vi "AddNextNode.vi"(8 "error in (no error)":errorcluster, 10 "Palette Name(Next)":string, 11 "VI Ref":refnum<vi>) -> (0 "error out":errorcluster)   [LabVIEW 2014]
doc: "Select a node and invoke this QD plugin to add the new node next to the selected node and connect the wires. It also clean the wires between these two nodes.\n\nDefault Shortcut - [N]"
panel:
  in  "Undo Name":string="Quick Drop Keyboard Shortcut"
  # "Specify the name of the Undo transaction"
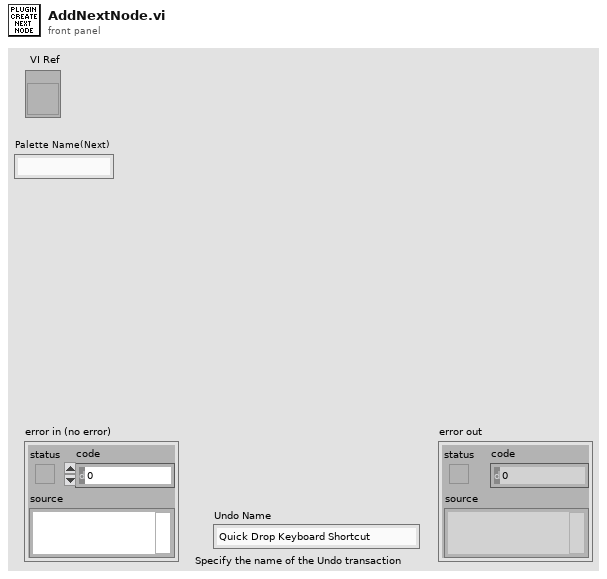
[diagram p1: front panel]
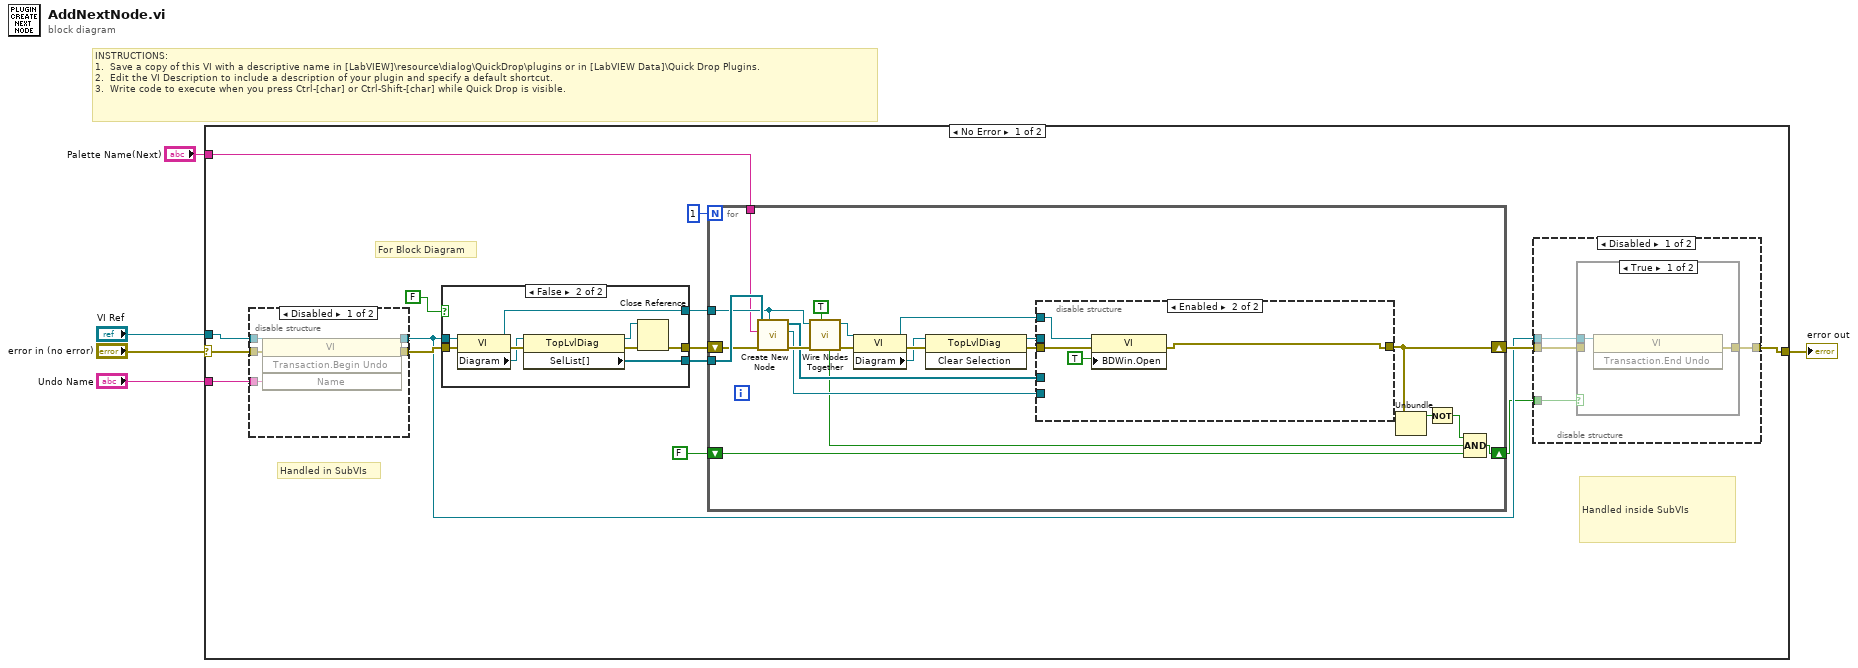
[diagram p0: block diagram]
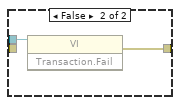
[diagram p2: hidden frame]
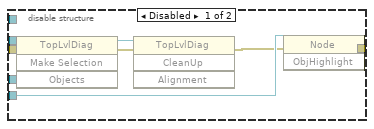
[diagram p5: hidden frame]
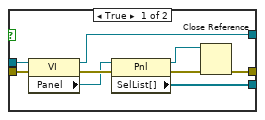
[diagram p6: hidden frame]
diagram:
  # "INSTRUCTIONS:\n1.  Save a copy of this VI with a descriptive name in [LabVIEW]\\resource\\dialog\\QuickDrop\\plugins or in [LabVIEW Data]\\Quick Drop Plugins.\n2.  Edit the VI Description to include a description of your plugin and specify a default shortcut. \n3.  Write code to execute when you press Ctrl-[char] or Ctrl-Shift-[char] while Quick Drop is visible."
  n1 = case shown="No Error" "error in (no error)" {
    selector: "error in (no error)" -> [w20 w88]
    tunnel: [w16 w88] -> w4
    tunnel: "VI Ref" -> [w19 _]
    tunnel: "Undo Name" -> [w18 _]
    tunnel: "Palette Name(Next)" -> [w6 _]
    frame No Error {
      # "Handled in SubVIs"
      # "For Block Diagram"
      # "Handled inside SubVIs"
      n2 = disable-structure shown="Disabled" {
        disable-tunnel: w20 -> [w34 w36]
        disable-tunnel: w19 -> [w33 w35]
        disable-tunnel: w18 -> [w32 _]
        disable-tunnel: [w31 w36] -> w17
        disable-tunnel: [w30 w35] -> w13
        frame Disabled {
          n3 = invoke class="VI" method="Transaction.Begin Undo"(reference=w33, error in=w34, "Name"=w32) -> (reference out=w30:refnum<vi>, error out=w31:errorcluster)  [unwired: 1 in, 2 out]
        }
        frame Enabled {
        }
      }
      n4 = case shown="False" FALSE {
        tunnel: w17 -> [w78 w87]
        tunnel: w13 -> [w77 w86]
        tunnel: [w72 w81] -> w15
        tunnel: [w71 w80] -> w9
        tunnel: [w70 w79] -> w8
        frame True {
          n5 = property class="VI"(reference=w77, error in=w78) -> (reference out=w70:refnum<vi>, error out=w76:errorcluster, "Panel"=w75:refnum<vi>)
          n6 = property class="Pnl"(reference=w75, error in=w76) -> (reference out=w73:refnum<vi>, error out=w74:errorcluster, "SelList[]"=w71:refnum<vi>[])
          n7 = Close Reference(reference=w73, error in (no error)=w74) -> (error out=w72:errorcluster)
        }
        frame False {
          n8 = property class="VI"(reference=w86, error in=w87) -> (reference out=w79:refnum<vi>, error out=w85:errorcluster, "Diagram"=w84:refnum<vi>)
          n9 = property class="TopLvlDiag"(reference=w84, error in=w85) -> (reference out=w82:refnum<vi>, error out=w83:errorcluster, "SelList[]"=w80:refnum<vi>[])
          n10 = Close Reference(reference=w82, error in (no error)=w83) -> (error out=w81:errorcluster)
        }
      }
      n11 = for {
        N: 1 -> [_]
        shift-right: [w51] -> w14
        shift-left: w15 -> [w53]
        shift-right: [w57] -> w11
        shift-left: FALSE -> [w38]
        tunnel: w9 -> [w54]
        tunnel: w8 -> [w52]
        tunnel: w6 -> [w41]
        n12 = call "Create New Node.vi"("VI Ref"=w52, "error in (no error)"=w53, "Palette String"=w41, "SelList[]"=w54) -> ("error out"=w56:errorcluster, "Node Refnum"=w50:refnum<vi>, "Array"=w42:refnum<vi>[])  [unwired: 5 in]
        n13 = call "Wire Nodes Together.vi"("Shift Pressed?"=TRUE, "error in (no error)"=w56, "VI Ref"=w52) -> ("error out"=w48:errorcluster, "dup VI"=w47:refnum<vi>, "Undo Fail?"=w39:bool)  [unwired: 6 in]
        n14 = property class="VI"(reference=w47, error in=w48) -> (reference out=w40:refnum<vi>, error out=w46:errorcluster, "Diagram"=w45:refnum<vi>)
        n15 = invoke class="TopLvlDiag" method="Clear Selection"(reference=w45, error in=w46) -> (reference out=w44:refnum<vi>, error out=w43:errorcluster)  [unwired: 1 in, 1 out]
        n16 = disable-structure shown="Enabled" {
          disable-tunnel: [w65 w66] -> w51
          disable-tunnel: w50 -> [w64 _]
          disable-tunnel: w44 -> [w63 _]
          disable-tunnel: w43 -> [w62 w67]
          disable-tunnel: w42 -> [w61 _]
          disable-tunnel: w40 -> [_ w68]
          frame Disabled {
            n17 = invoke class="TopLvlDiag" method="Make Selection"(reference=w63, error in=w62, "Objects"=w61) -> (reference out=w58:refnum<vi>, error out=w60:errorcluster)  [unwired: 1 in, 2 out]
            n18 = invoke class="TopLvlDiag" method="CleanUp"(reference=w58, error in=w60) -> (error out=w59:errorcluster)  [unwired: 2 in, 3 out]
            n19 = invoke class="Node" method="ObjHighlight"(reference=w64, error in=w59) -> (error out=w65:errorcluster)  [unwired: 1 in, 2 out]
          }
          frame Enabled {
            n20 = property class="VI"(reference=w68, error in=w67, "BDWin.Open"=TRUE ("Block Diagram Window:Open")) -> (error out=w66:errorcluster)  [unwired: 1 out]
          }
        }
        n21 = Unbundle(w51) -> ("status"=w49:bool)  [unwired: 2 out]
        n22 = Not(x=w49) -> (.not. x?=w37:bool)
        n23 = Compound Arithmetic op=AND(w37, w39, w38) -> (w57:bool)
      }
      n24 = disable-structure shown="Disabled" {
        disable-tunnel: [w24 w29] -> w16
        disable-tunnel: w14 -> [w23 w29]
        disable-tunnel: w13 -> [w22 _]
        disable-tunnel: w11 -> [w21 _]
        frame Disabled {
          n25 = case shown="True" w21 {
            tunnel: w22 -> [w25 w27]
            tunnel: [w26 w28] -> w24
            tunnel: w23 -> [_ _]
            frame True {
              n26 = invoke class="VI" method="Transaction.End Undo"(reference=w25) -> (error out=w26:errorcluster)  [unwired: 2 in, 2 out]
            }
            frame False {
              n27 = invoke class="VI" method="Transaction.Fail"(reference=w27) -> (error out=w28:errorcluster)  [unwired: 2 in, 2 out]
            }
          }
        }
        frame Enabled {
        }
      }
    }
    frame Error {
    }
  }
  "error out" <- w4
